vi "GetSource.vi"(9 "Error in":errorcluster) -> (1 "Source":string)   [LabVIEW 2017, in "GPError.lvlib"]
doc: "Returns the source part of the Source field of <B>Error in</B>.\n\nAny timestamp and custom error descriptions are stripped from <B>Source</B>. For appended errors the source from the primary error/warning is returned only.\n\nThis VI is inlined.\n\nSteen Schmidt\nGPower\n14/11 2014"
uses:
  GPError.lvlib
panel:
  # "Copyright © 2014\nGPower\nSee enclosed license file for terms and conditions"
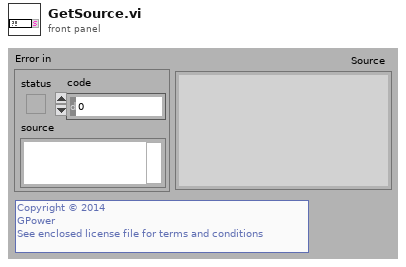
[diagram p1: front panel]
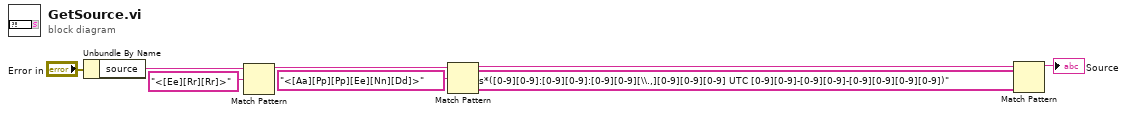
[diagram p0: block diagram]
diagram:
  n1 = Unbundle By Name("Error in") -> ("source"=w6:string)
  n2 = Match Pattern(string=w6, regular expression="<[Ee][Rr][Rr]>") -> (before substring=w4:string)  [unwired: 1 in, 3 out]
  n3 = Match Pattern(string=w4, regular expression="<[Aa][Pp][Pp][Ee][Nn][Dd]>") -> (before substring=w2:string)  [unwired: 1 in, 3 out]
  n4 = Match Pattern(string=w2, regular expression="\\s*([0-9][0-9]:[0-9][0-9]:[0-9][0-9][\\.,][0-9][0-9][0-9] UTC [0-9][0-9]-[0-9][0-9]-[0-9][0-9][0-9][0-9])" ("time format string (%c)")) -> (before substring=→"Source":string)  [unwired: 1 in, 3 out]
